vi "Configure.vi"(0 "WaveformAddressSpace in":refnum<class "WaveformAddressSpace.lvclass">, 5 "oclk_freq":u32, 7 "oclk_mult":u32, 9 "UnderflowMargin":u32=3) -> (4 "WaveformAddressSpace out":refnum<class "WaveformAddressSpace.lvclass">)   [LabVIEW 2017, in "WaveformAddressSpace.lvclass"]
uses:
  WaveformAddressSpace.lvclass
  WaveformAddressSpace.lvclass/WaveformAddressSpace.ctl
  <vilib>/rvi/DataTransferAndStorage/Container/Common/niFpgaContainerExecOnDevCompGetState.vi
  <vilib>/rvi/Emulation/niFpgaEmulationIsFPGAContextNoSignature.vi
  <vilib>/rvi/DataTransferAndStorage/Container/Common/niFpgaContainerGetUniqueNameForEmu.vi
  <vilib>/rvi/Memory/Memory_Emulation/niFpgaMemoryEmulationCacheClearOnFirstRun.vi
  <vilib>/rvi/Memory/Memory_Emulation/nirvimemoryEmulationManagerCache_MakeExclusive.vi
  <vilib>/rvi/Memory/Memory_Emulation/niFpgaMemoryEmulationValidateCache.vi
  <vilib>/rvi/Memory/Memory_Emulation/nirvimemoryEmulationManagerCache_InsertValue.vi
  <vilib>/Utility/error.llb/Clear Errors.vi
  <vilib>/rvi/Memory/Memory_Emulation/nirvimemoryEmulationManagerCache_ReleaseExclusive.vi
  <vilib>/rvi/Memory/Memory_Emulation/nirvimemoryEmulationManagerCache_GetValue.vi
  <vilib>/rvi/Memory/Memory_Emulation/nirvimemoryEmulationManagerCache_SetValue.vi
  <vilib>/rvi/Emulation/niFpgaProcessEmulError.vi
  <vilib>/rvi/Emulation/niFpgaSctlEmulationGetInTimedLoop.vi
  <vilib>/rvi/DataTransferAndStorage/Container/XNode/niFpgaContainer.xnode
  <vilib>/rvi/DataTransferAndStorage/Register/Emulation/niFpgaRegisterEmulationRefIn.vi
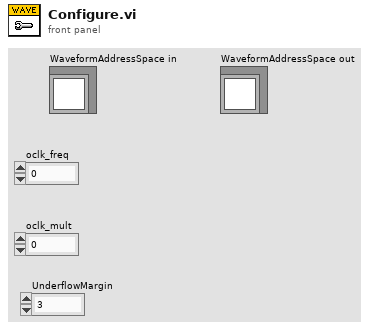
[diagram p1: front panel]
types:
  T1 = typedef "WaveformAddressSpace.lvclass/Registers.ctl" = cluster{"oclk_freq":refnum<k21>, "data_rate":refnum<k21>, "oclk_div":refnum<k21>, "oclk_mult":refnum<k21>, "AcquisitionType":refnum<k21>, "SamplesPerChan":refnum<k21>, "NumberOfChannels":refnum<k21>, "stop":refnum<k21>, "FIFO":refnum<k21>, "FirstRead":refnum<k21>, "ErrorCode":refnum<k21>, "ChannelCount":refnum<k21>, "Finished":refnum<k21>, "DMA_FIFO_Full":refnum<k21>, "ModuleUnderflow":refnum<k21>, "ConfigReadyIRQ":refnum<k21>, "ConfigReadyAck":refnum<k21>, "SynchStartIRQ":refnum<k21>, "SynchStartAck":refnum<k21>, "UnderflowCount":refnum<k21>, "FirstReadReset":refnum<k21>}
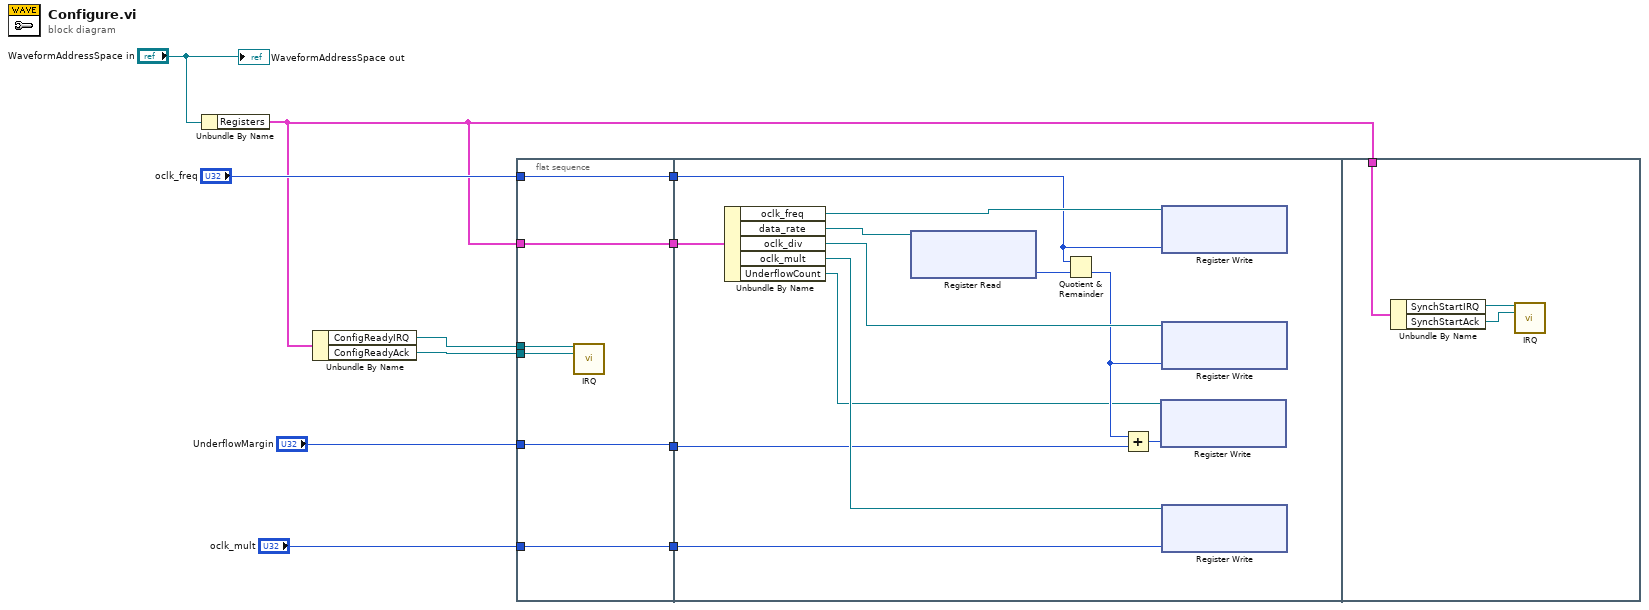
[diagram p0: block diagram]
diagram:
  n1 = Unbundle By Name("WaveformAddressSpace in") -> ("Registers"=w2:T1)
  n2 = Unbundle By Name(w2) -> ("ConfigReadyIRQ"=w6:refnum<k21>, "ConfigReadyAck"=w5:refnum<k21>)
  n3 = flat-sequence {
    tunnel: "oclk_mult" -> [w15]
    tunnel: "oclk_freq" -> [w16]
    tunnel: w2 -> [w17]
    tunnel: [w17] -> w9
    tunnel: [w16] -> w8
    tunnel: [w15] -> w7
    tunnel: w6 -> [w14]
    tunnel: w5 -> [w13]
    tunnel: [w12] -> w4
    tunnel: "UnderflowMargin" -> [w12]
    tunnel: w9 -> [w29]
    tunnel: w8 -> [w26]
    tunnel: w7 -> [w22]
    tunnel: w4 -> [w19]
    tunnel: w2 -> [w32]
    frame #0 {
      n4 = call "IRQ.vi"("IRQ"=w14, "Ack"=w13) -> ()  [unwired: 14 in]
    }
    frame #1 {
      n5 = Unbundle By Name(w29) -> ("oclk_freq"=w28:refnum<k21>, "data_rate"=w27:refnum<k21>, "oclk_div"=w24:refnum<k21>, "oclk_mult"=w23:refnum<k21>, "UnderflowCount"=w20:refnum<k21>)
      n6 = xnode ("Register Read")("Register In"=w27) -> ("Data"=w25:u32)  [unwired: 1 out]
      n7 = Quotient & Remainder(x=w26, y=w25) -> (floor(x/y)=w21:u32)  [unwired: 1 out]
      n8 = Add(x=w21, y=w19) -> (x+y=w18:u32)
      n9 = xnode ("Register Write")("Data"=w18, "Register In"=w20) -> ()  [unwired: 1 out]
      n10 = xnode ("Register Write")("Data"=w26, "Register In"=w28) -> ()  [unwired: 1 out]
      n11 = xnode ("Register Write")("Data"=w21, "Register In"=w24) -> ()  [unwired: 1 out]
      n12 = xnode ("Register Write")("Data"=w22, "Register In"=w23) -> ()  [unwired: 1 out]
    }
    frame #2 {
      n13 = Unbundle By Name(w32) -> ("SynchStartIRQ"=w31:refnum<k21>, "SynchStartAck"=w30:refnum<k21>)
      n14 = call "IRQ.vi"("IRQ"=w31, "Ack"=w30) -> ()  [unwired: 14 in]
    }
  }
  "WaveformAddressSpace out" <- "WaveformAddressSpace in"
